vi "GlobalVaribles.vi"() -> ()   [LabVIEW 2019]
uses:
  <userlib>/LaguerreDeconLib/DeconEngineClass/LaguerreDeconEngineClass.lvclass
panel:
  in  "LaguerreDeconEngine":refnum<class "LaguerreDeconEngineClass.lvclass">
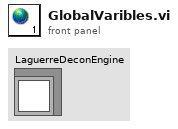
[diagram p1: front panel]
diagram:
